vi "Image gray scale 04.vi"() -> ()   [LabVIEW 2018]
uses:
  <vilib>/Math Plots/3D Math Plots/3D Surface/3D Surface XCtrl/3D Surface.xctl
  <vilib>/Instr/_visa.llb/VISA Configure Serial Port (Instr).vi
  <vilib>/Math Plots/3D Math Plots/3D Surface/3D Surface Datatype/Public/Plot Helper (Matrix).vi
  <vilib>/Math Plots/3D Math Plots/3D Surface/3D Surface Datatype/3D Surface Datatype.lvclass
panel:
  in  "탭 컨트롤":enum32{"2D", "3D"}(tab)
  out "Temperature":dbl[][](graph)
  out "최대온도":dbl
  out "웨이브폼 차트":dbl(graph)
  out "3D Surface 2":refnum<class "3D Plot Datatype.lvclass">[](xcontrol) caption="3D 표면"
  in  "길이":i32=1
  in  "인덱스 (열)":i32
  in  "열 화상 촬영":path
  in  "stop 4":bool
  in  "stop 3":bool
  in  "VISA resource name":refnum<visa-resource-name>="COM6"
  in  "Stop":bool
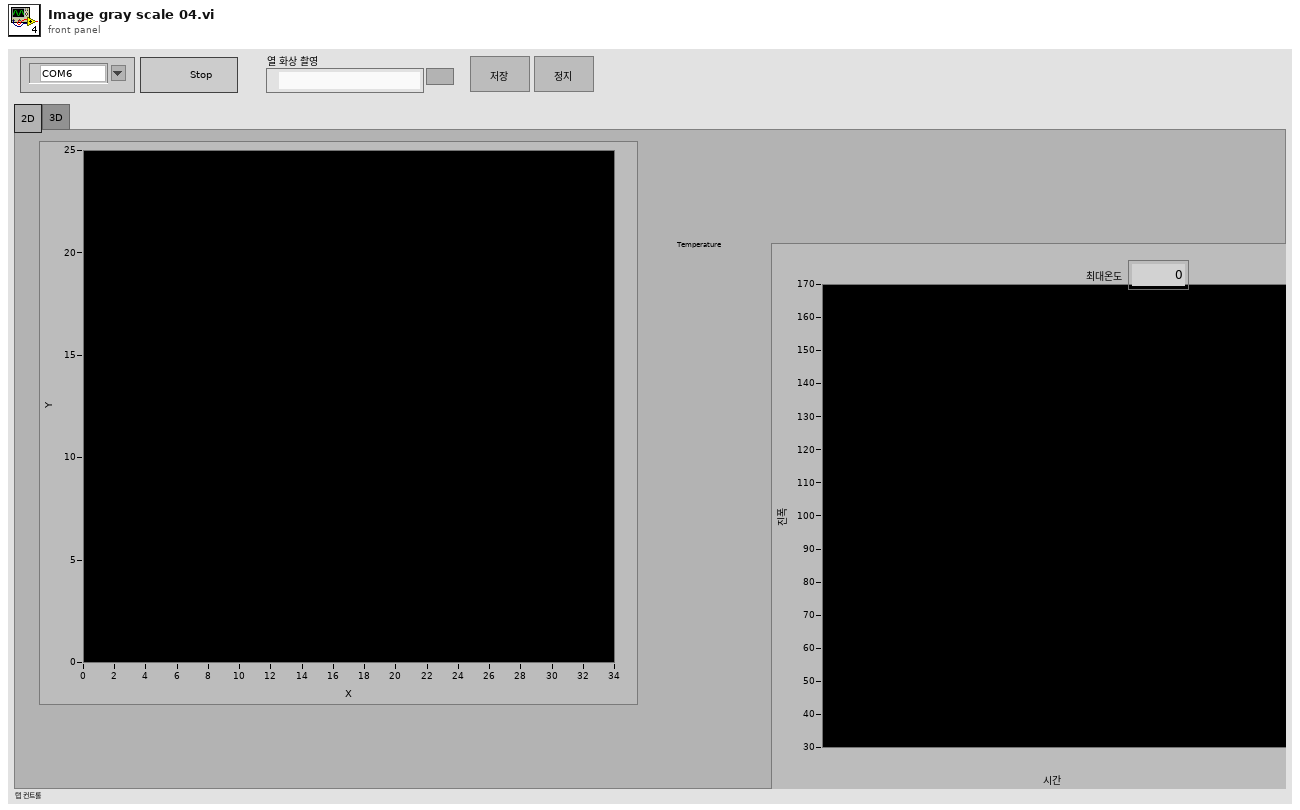
[diagram p1: front panel]
types:
  T1 = typedef "Image Type" = u32
  T2 = typedef "IMAQ Image.ctl" = refnum<image>
  T3 = typedef "IMAQ AVI2 Refnum.ctl" = refnum<k20>
  T4 = typedef "imagedata.ctl" = cluster{"image type":i32, "image depth":i32, "image":u8[], "mask":u8[], "colors":u32[], "Rectangle":cluster{"left":i16, "top":i16, "right":i16, "bottom":i16}}
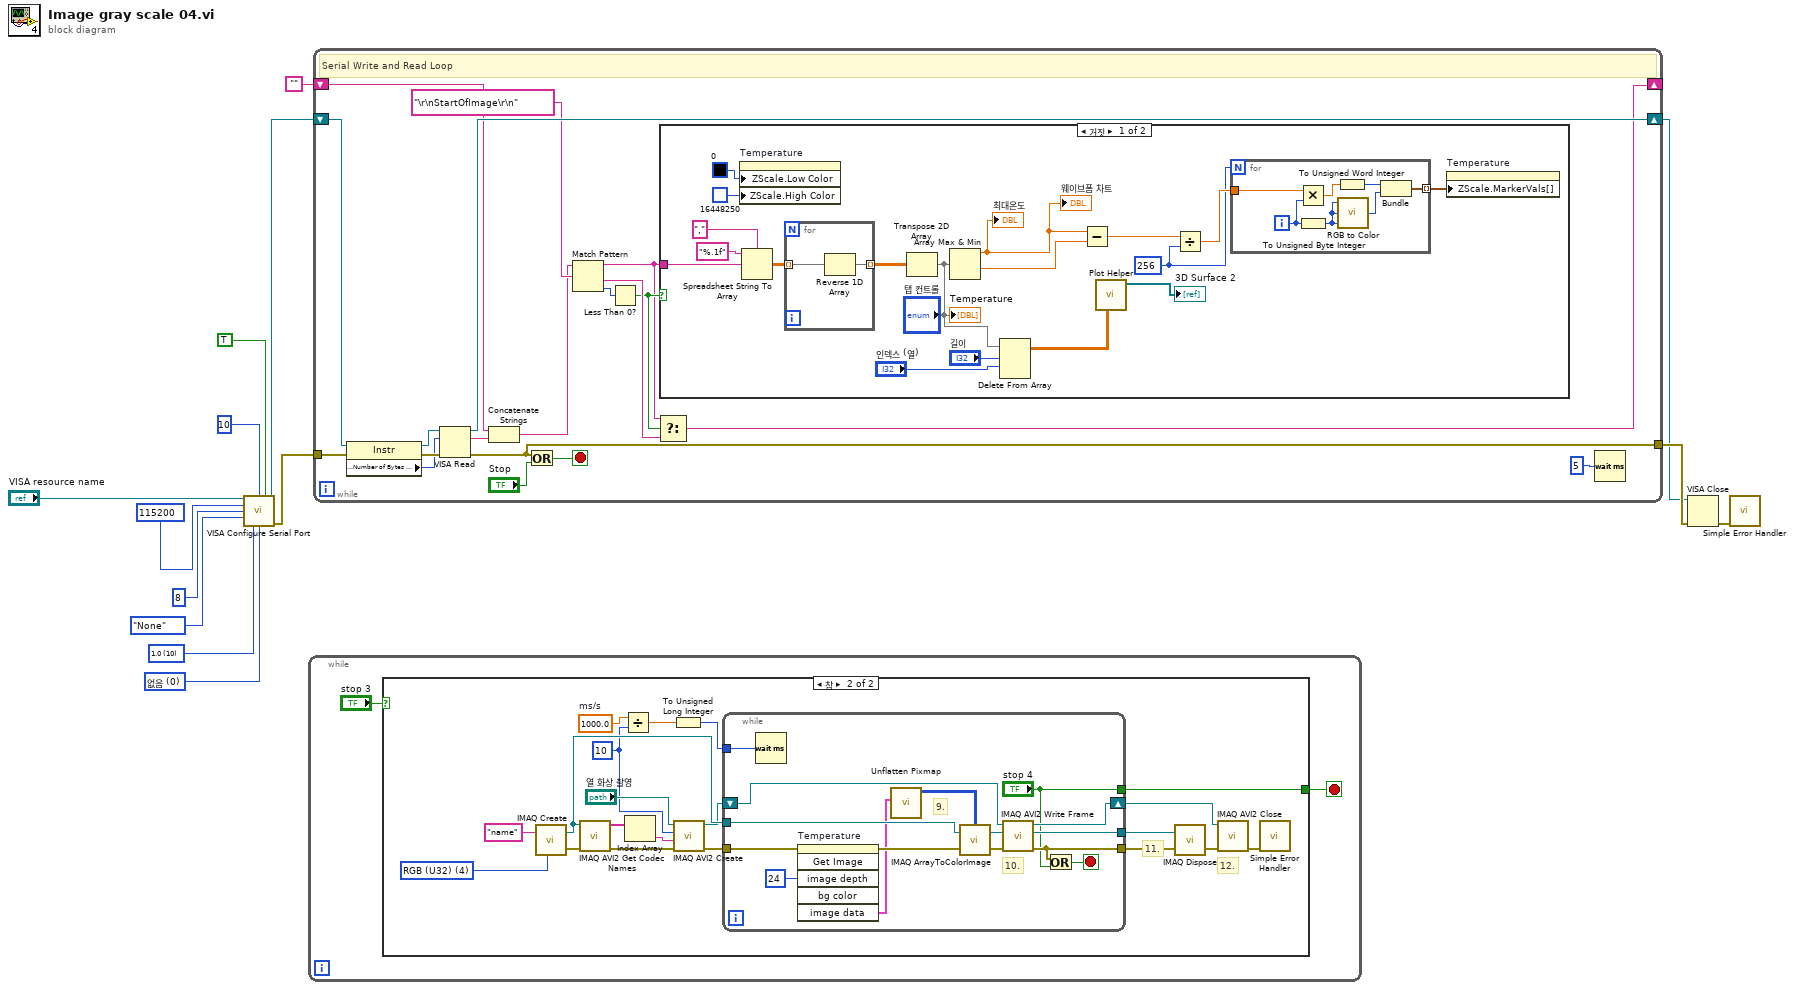
[diagram p0: block diagram]
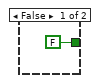
[diagram p2: hidden frame]
diagram:
  w1 = u16 0 items=["없음", "XON/XOFF", "RTS/CTS", "XON/XOFF & RTS/CTS", "DTR/DSR", "XON/XOFF & DTR/DSR"] ("flow control (0:none)")
  w2 = u16 10 items=["1.0"=10, "1.5"=15, "2.0"=20] ("stop bits (10: 1 bit)")
  n1 = call-poly "VISA Configure Serial Port"("VISA resource name"="VISA resource name", "termination char\n(0xA = '\\n' = LF)"=u8 10 ("Termination Character"), "Enable Termination\nChar (T)"=TRUE ("End Read on Termination Character?"), "baud rate (9600)"=u32 115200, "data bits (8)"=u16 8, "parity (0:none)"=enum16{"None", "Odd", "Even", "Mark", "Space"}."None", "stop bits (10: 1 bit)"=w2, "flow control (0:none)"=w1) -> ("VISA resource name out"=w8:refnum<visa-resource-name>, "error out"=w7:errorcluster)  [unwired: 2 in, 4 out]
  n2 = while {
    stop <- w15 stop-if-true
    n3 = case shown="참" "stop 3" {
      tunnel: [FALSE ("stop") w19] -> w15
      frame False {
      }
      frame True {
        w18 = u32 10 ("Frames/ Per Second")
        w22 = 1000.0  # ms/s
        w20 = T1 4 items=["Grayscale (U8)", "Grayscale (I16)", "Grayscale (SGL)", "Complex (CSG)", "RGB (U32)", "HSL (U32)", "RGB (U64)", "Grayscale (U16)"] ("Image Type")
        # "12."
        # "11."
        n4 = call "IMAQ Create"("Image Name"="name", "Image Type"=w20) -> ("New Image"=w32:T2, "error out"=w31:errorcluster)  [unwired: 3 in]
        n5 = call "IMAQ AVI2 Get Codec Names"("error in (no error)"=w31, "Image"=w32) -> ("error out"=w30:errorcluster, "Codec Names"=w34:string[])  [unwired: 8 in]
        n6 = Divide(x=w22, y=w18) -> (x/y=w36:dbl)
        n7 = Index Array(array=w34) -> (element=w35:string)  [unwired: 1 in]
        n8 = To Unsigned Long Integer(number=w36) -> (unsigned 32bit integer=w37:u32)
        n9 = call "IMAQ AVI2 Create"("error in (no error)"=w30, "Codec"=w35, "Frames Per Second"=w18, "AVI Path"="열 화상 촬영") -> ("error out"=w33:errorcluster, "AVI Refnum"=w29:T3)  [unwired: 6 in]
        n10 = while {
          tunnel: w32 -> [w46]
          tunnel: w33 -> [w41]
          tunnel: [w50] -> w23
          tunnel: [w47] -> w24
          shift-right: [w51] -> w25
          shift-left: w29 -> [w52]
          tunnel: w37 -> [w49]
          tunnel: ["stop 4"] -> w19
          stop <- w48 stop-if-true
          # "10."
          # "9."
          n11 = Wait (ms)(milliseconds to wait=w49) -> ()  [unwired: 1 out]
          n12 = invoke on="Temperature" class="IntGraph (엄격한)" method="Get Image"(error in=w41, "image depth"=24 ("Image Depth")) -> (error out=w40:errorcluster, "image data"=w39:T4)  [unwired: 4 in, 4 out]
          n13 = call <vilib>:"Unflatten Pixmap.vi"("image data"=w39) -> ("24-bit pixmap"=w43:u32[][])  [unwired: 4 in, 6 out]
          n14 = call "IMAQ ArrayToColorImage"("Image Pixels (U32)"=w43, "Image"=w46, "error in (no error)"=w40) -> ("Image Out"=w45:T2, "error out"=w44:errorcluster)  [unwired: 2 in]
          n15 = call "IMAQ AVI2 Write Frame"("error in (no error)"=w44, "Image"=w45, "AVI Refnum"=w52) -> ("error out"=w47:errorcluster, "Image Out (duplicate)"=w50:T2, "AVI Refnum (duplicate)"=w51:T3)  [unwired: 6 in]
          n16 = Or(x=w47, y="stop 4") -> (x .or. y?=w48:bool)
        }
        n17 = call "IMAQ Dispose"("Image"=w23, "error in (no error)"=w24) -> ("error out"=w26:errorcluster)  [unwired: 4 in]
        n18 = call "IMAQ AVI2 Close"("error in (no error)"=w26, "AVI Refnum"=w25) -> ("error out"=w27:errorcluster)  [unwired: 9 in]
        n19 = call <vilib>:"Simple Error Handler.vi"("error in (no error)"=w27) -> ()  [unwired: 4 in, 5 out]
      }
    }
  }
  n20 = while {
    shift-right: [w66] -> w10
    shift-left: w8 -> [w68]
    tunnel: w7 -> [w64]
    tunnel: [w60] -> w11
    shift-right: [w53] -> _
    shift-left: "" -> [w62]
    stop <- w70 stop-if-true
    # "Serial Write and Read Loop"
    n21 = property class="Instr"(reference=w68, error in=w64) -> (reference out=w67:refnum<visa-resource-name>, error out=w65:errorcluster, "Serial Settings:Number of Bytes at Serial Port"=w63:u32)
    n22 = VISA Read(VISA resource name=w67, byte count=w63, error in (no error)=w65) -> (VISA resource name out=w66:refnum<visa-resource-name>, read buffer=w61:string, error out=w60:errorcluster)  [unwired: 1 out]
    n23 = Concatenate Strings(w62, w61) -> (w58:string)
    n24 = Or(x=w60, y="Stop") -> (x .or. y?=w70:bool)
    n25 = Match Pattern(string=w58, regular expression="\r\nStartOfImage\r\n") -> (before substring=w54:string, after substring=w56:string, offset past match=w57:i32)  [unwired: 1 in, 1 out]
    n26 = Less Than 0?(x=w57) -> (x < 0?=w55:bool)
    n27 = Select(t=w54, s=w55, f=w56) -> (s? t:f=w53:string)
    n28 = case shown="거짓" w55 {
      tunnel: w54 -> [w88 _]
      frame False {
        w79 = 256
        n29 = property on="Temperature" class="IntGraph (엄격한)"("ZScale.Low Color"=u32 0, "ZScale.High Color"=u32 16448250) -> ()  [unwired: 2 in, 2 out]
        n30 = Spreadsheet String To Array(delimiter (Tab)=",", format string="%.1f", spreadsheet string=w88) -> (array=w86:dbl[][])  [unwired: 1 in]
        n31 = for {
          tunnel: w86 -> [w98] mode=indexing
          tunnel: [w97] -> w85 mode=indexing
          n32 = Reverse 1D Array(array=w98) -> (reversed array=w97:dbl[])
        }
        n33 = Transpose 2D Array(2D array=w85) -> (transposed array=w72:dbl[][])
        "Temperature" <- w72
        n34 = Array Max & Min(array=w72) -> (max value=w78:dbl, min value=w77:dbl)  [unwired: 2 out]
        "최대온도" <- w78
        "웨이브폼 차트" <- w78
        n35 = Delete From Array(array=w72, length="길이", index (row)="인덱스 (열)") -> (array with subset deleted=w75:dbl[][])  [unwired: 1 in, 1 out]
        n36 = Subtract(x=w78, y=w77) -> (x-y=w82:dbl)
        n37 = call-poly <vilib>:"Plot Helper.vi"("z matrix"=w75) -> ("3D Plot lvclass Array out"=→"3D Surface 2":refnum<class "3D Plot Datatype.lvclass">[])  [unwired: 5 in, 5 out]
        n38 = Divide(x=w82, y=w79) -> (x/y=w83:dbl)
        n39 = for {
          N: w79 -> [_]
          tunnel: [w94] -> w84 mode=indexing
          tunnel: w83 -> [w93]
          i -> [w92]
          n40 = Multiply(x=w93, y=w92) -> (x*y=w91:dbl)
          n41 = To Unsigned Byte Integer(number=w92) -> (unsigned 8bit integer=w96:u8)
          n42 = To Unsigned Word Integer(number=w91) -> (unsigned 16bit integer=w90:u16)
          n43 = call <vilib>:"RGB to Color.vi"("B"=w96, "G"=w96, "R"=w96) -> ("Color"=w95:u32)
          n44 = Bundle(w90, "Color"=w95) -> (w94:cluster{u16, "Color":u32})  [unwired: 1 in]
        }
        n45 = property on="Temperature" class="IntGraph (엄격한)"("ZScale.MarkerVals[]"=w84) -> ()  [unwired: 2 in, 2 out]
      }
      frame True {
      }
    }
    n46 = Wait (ms)(milliseconds to wait=u32 5) -> ()  [unwired: 1 out]
  }
  n47 = VISA Close(VISA resource name=w10, error in (no error)=w11) -> (error out=w12:errorcluster)
  n48 = call <vilib>:"Simple Error Handler.vi"("error in (no error)"=w12) -> ()  [unwired: 1 in, 8 out]
